vi "test1-TestModuleStatusVI.vi"(8 "error in (no error)":errorcluster, 11 "TestCase in":refnum<class "testcase-CSMManagementAPI.lvclass">) -> (0 "error out":errorcluster, 3 "TestCase out":refnum<class "testcase-CSMManagementAPI.lvclass">)   [LabVIEW 2017, in "testcase-CSMManagementAPI.lvclass"]
uses:
  testcase-CSMManagementAPI.lvclass
  src/user.lib/_NEVSTOP/Communicable State Machine(CSM)/_Support/Typedef/_CSM_MODE.ctl
  src/user.lib/_NEVSTOP/Communicable State Machine(CSM)/AdvanceAPI/CSM - Revert Arguments-Safe String.vi
  src/user.lib/_NEVSTOP/Communicable State Machine(CSM)/AdvanceAPI/CSM - Make String Arguments Safe.vi
  src/user.lib/_NEVSTOP/Communicable State Machine(CSM)/AdvanceAPI/CSM - Break Down Multiple States String.vi
  src/user.lib/_NEVSTOP/Communicable State Machine(CSM)/AdvanceAPI/CSM - Compact Multiple States.vi
  src/user.lib/_NEVSTOP/Communicable State Machine(CSM)/AdvanceAPI/CSM - Keywords.vi
  src/user.lib/_NEVSTOP/Communicable State Machine(CSM)/_Shared/Trim Single-line Text.vi
  <vilib>/addons/_JKI Toolkits/VI Tester/TestCase.llb/TestCase.lvclass
  src/user.lib/_NEVSTOP/Communicable State Machine(CSM)/Communicable State Machine.lvlib
  src/user.lib/_NEVSTOP/Communicable State Machine(CSM)/_Support/Typedef/_CSM_List Module Scope.ctl
  CSM/CSM-Testcase.lvlib
  C:/Program Files (x86)/National Instruments/LabVIEW 2017/vi.lib/addons/_JKI Toolkits/VI Tester/TestCase.llb/TestCase.lvclass
panel:
  out "State History":string
  out "LoopCount":i32
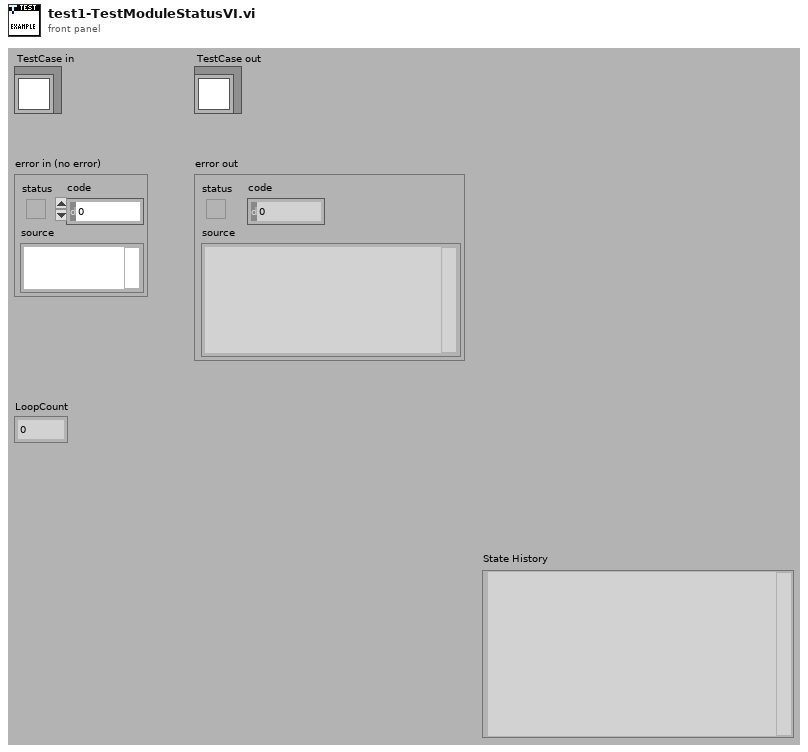
[diagram p1: front panel]
types:
  T1 = typedef "Communicable State Machine.lvlib/_CSM_MODE.ctl" = enum16{"Not Exist", "Stand Alone", "CSM", "Worker", "Worker Agent", "Chain Node", "Chain"}
  T2 = cluster{"CSM Name (Dup)":string, "Mode":T1, "#Nodes":i32}[]
  T3 = typedef "Communicable State Machine.lvlib/_CSM_List Module Scope.ctl" = enum16{"Normal", "System Only", "All"}
  T4 = enum32{"Invalid", "Standard", "Closed", "Hidden", "Minimized", "Maximized"}
  T5 = enum32{"invalid app kind", "Development System", "Run Time System", "Student Edition", "Embedded LabVIEW", "Evaluation", "Custom"}
  T6 = typedef "Communicable State Machine.lvlib/_CSM_Response Source Message.ctl" = cluster{"‘State":string, "’Arguments":string, "’Error":errorcluster}
  T7 = cluster{"Current VI Reference":refnum<vi>, "Close Panel on Exit?":bool}
  T8 = cluster{"Core":cluster{"Current VI Reference":refnum<vi>, "Close Panel on Exit?":bool}, "Your Boolean data":bool, "Your string data":string, "Module Status":cluster{"CSM Name (Dup)":string, "Mode":T1, "#Nodes":i32}}
  T9 = cluster{"CSM Name (Dup)":string, "Mode":T1, "#Nodes":i32}
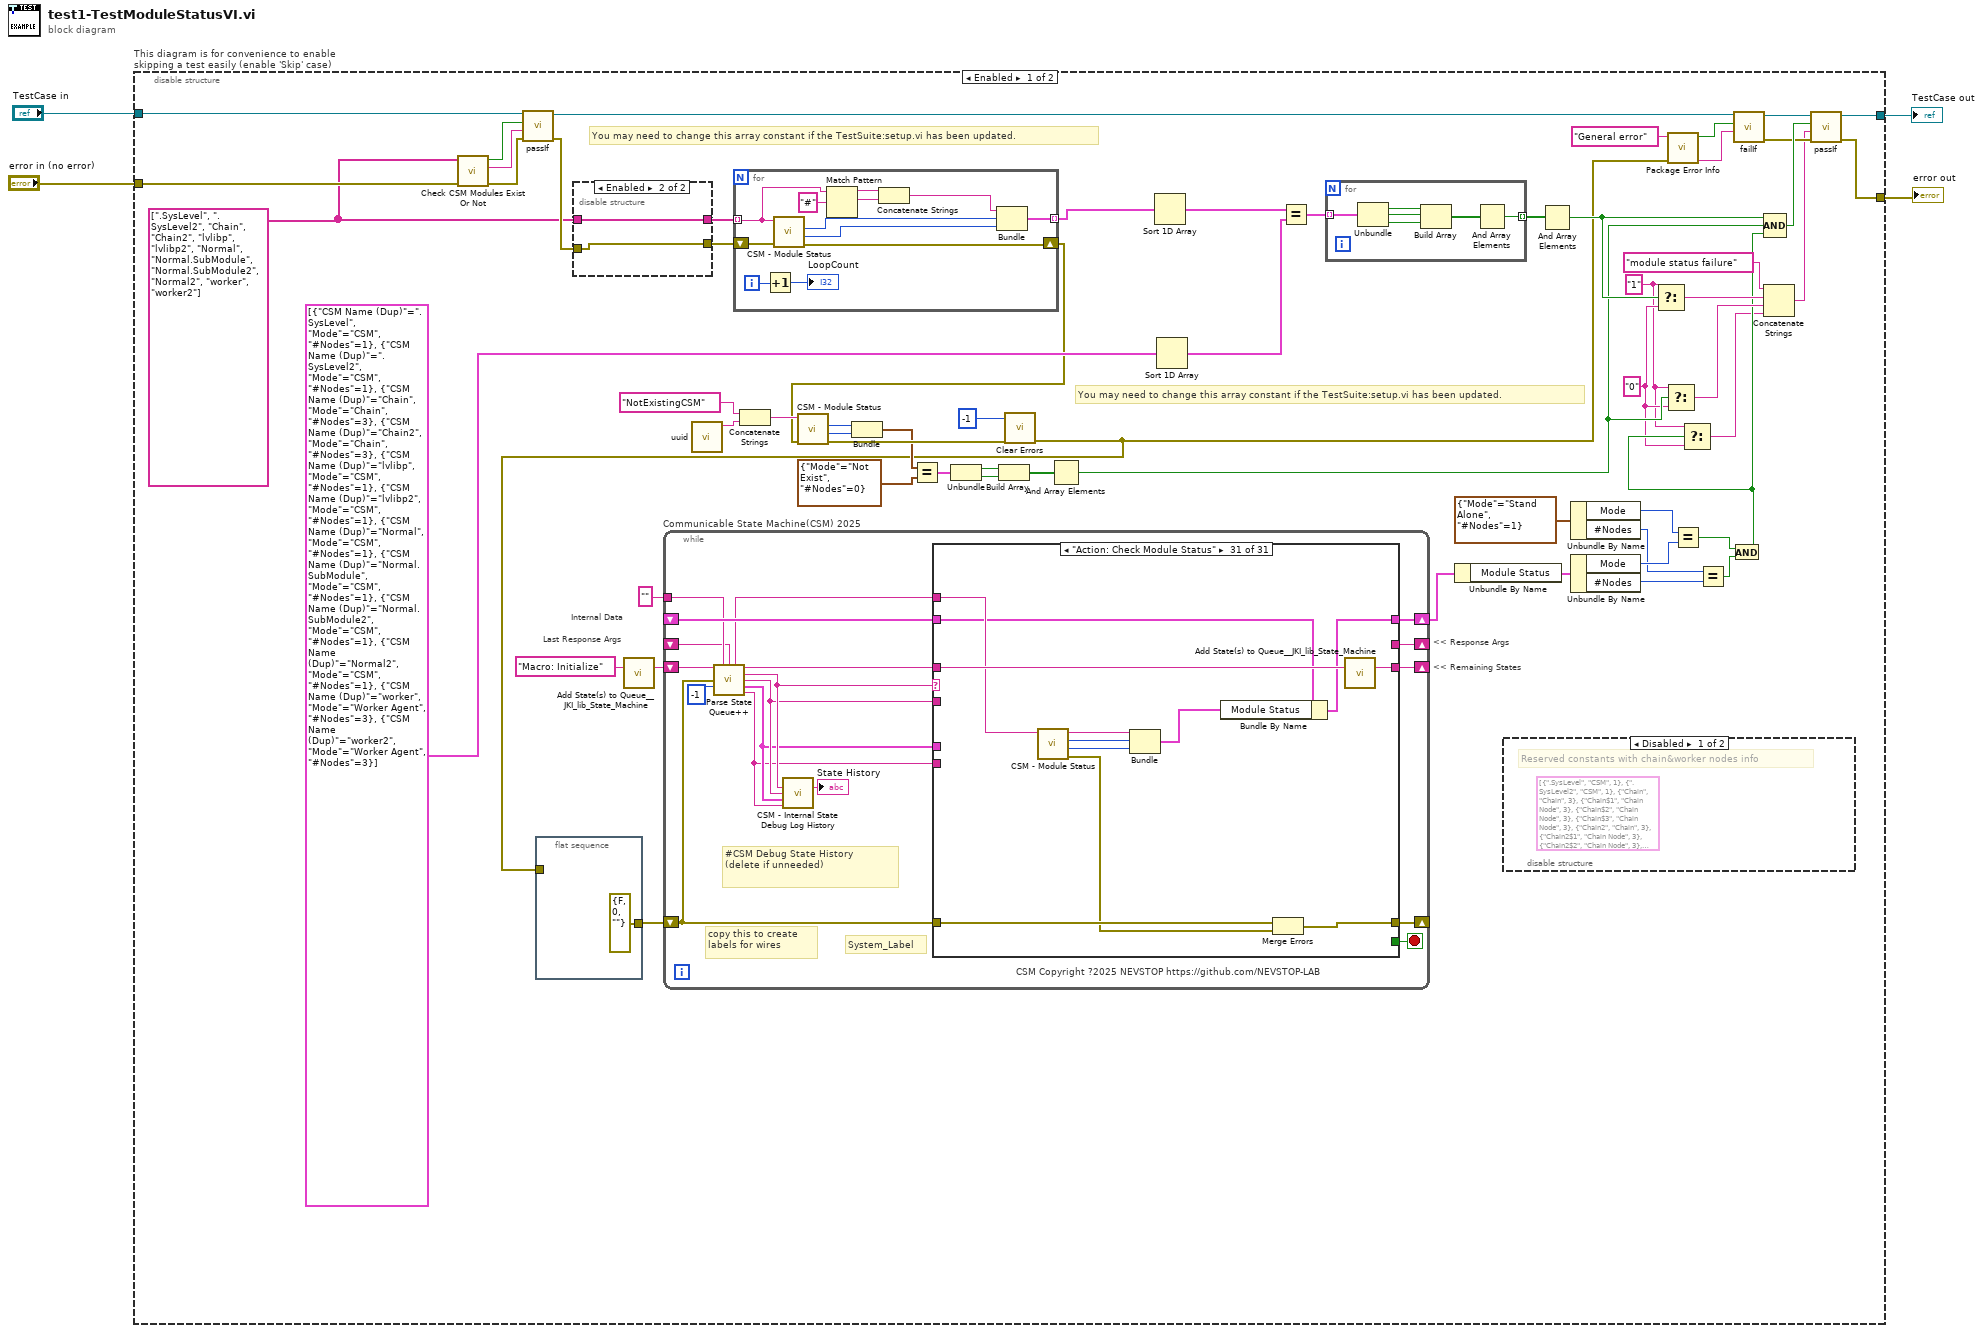
[diagram p0: block diagram]
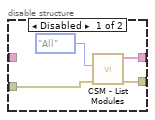
[diagram p3: hidden frame]
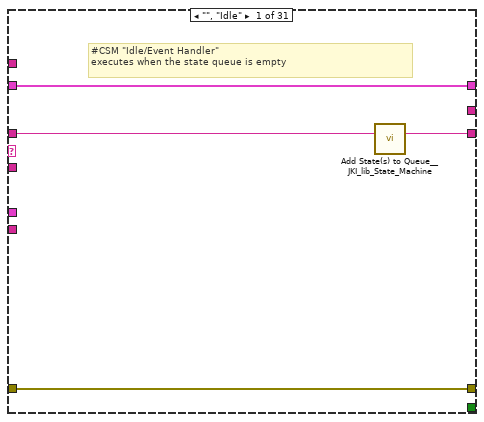
[diagram p4: hidden frame]
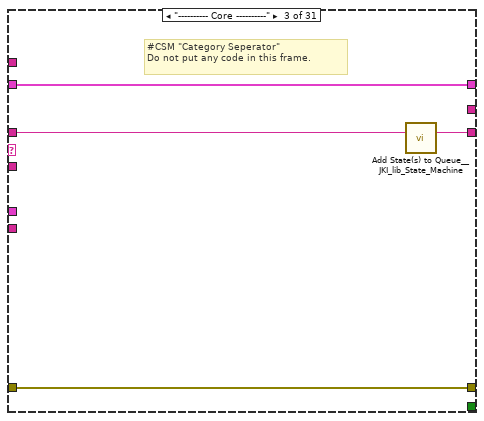
[diagram p6: hidden frame]
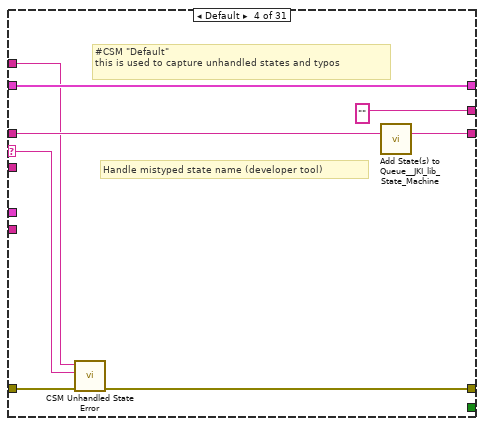
[diagram p7: hidden frame]
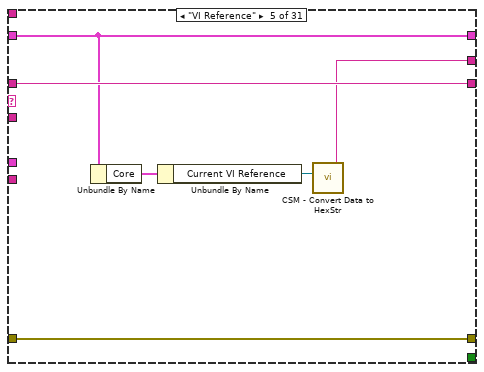
[diagram p8: hidden frame]
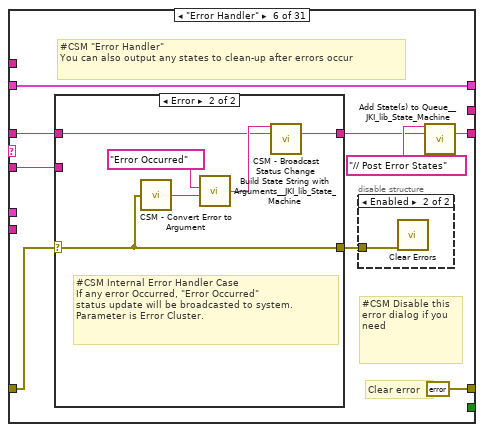
[diagram p9: hidden frame]
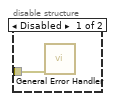
[diagram p10: hidden frame]
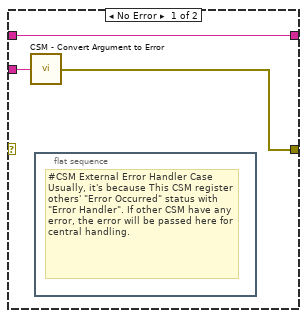
[diagram p11: hidden frame]
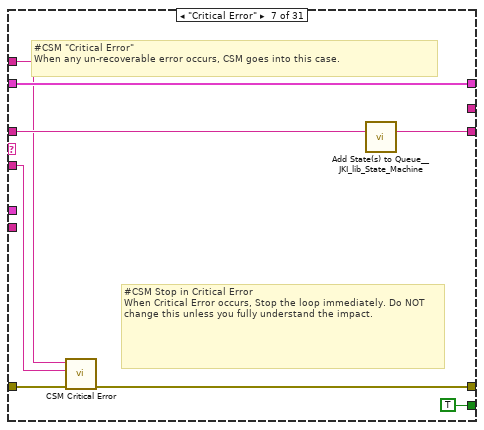
[diagram p12: hidden frame]
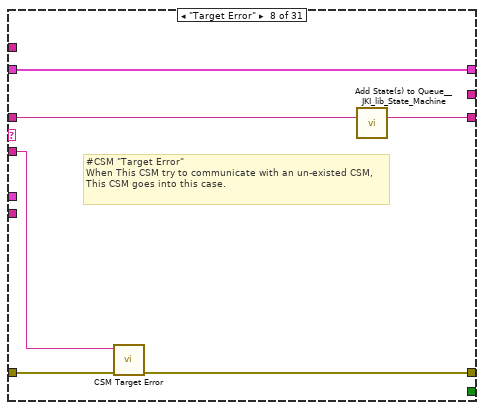
[diagram p13: hidden frame]
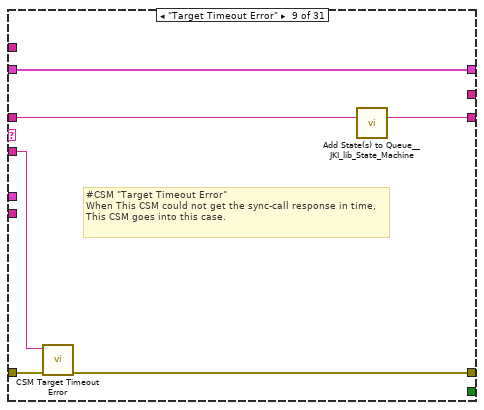
[diagram p14: hidden frame]
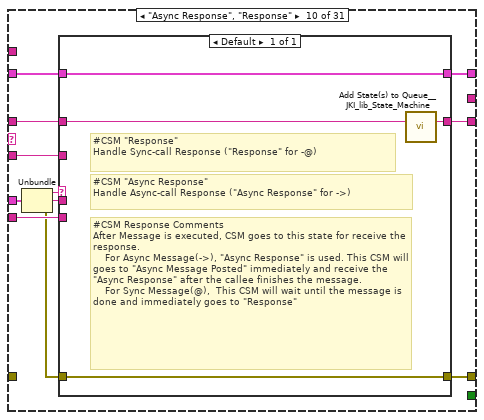
[diagram p15: hidden frame]
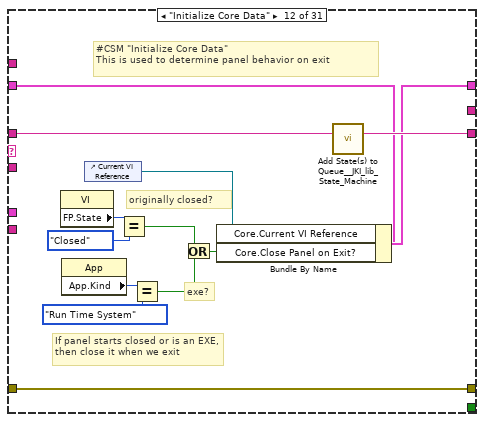
[diagram p17: hidden frame]
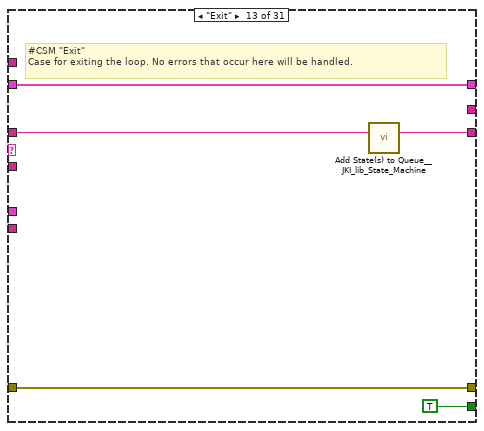
[diagram p18: hidden frame]
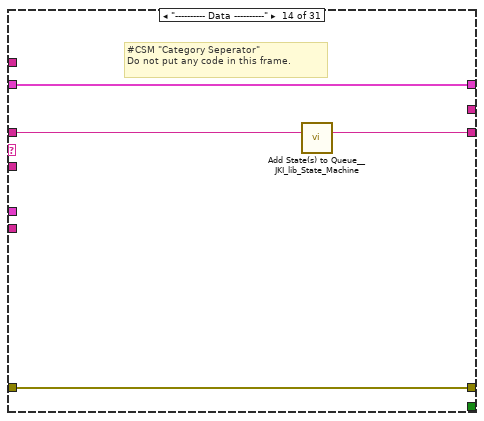
[diagram p19: hidden frame]
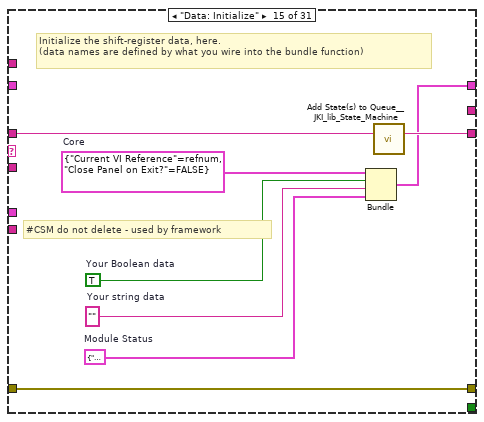
[diagram p20: hidden frame]
diagram:
  n1 = disable-structure "This diagram is for convenience to enable skipping a test easily (enable 'Skip' case)" shown="Enabled" {
    disable-tunnel: "TestCase in" -> [w26 w383]
    disable-tunnel: [w64 w381] -> w1
    disable-tunnel: [w63 w382] -> w3
    disable-tunnel: "error in (no error)" -> [w25 w380]
    frame Enabled {
      w11 = "0" ("f")
      w10 = "1"
      w5 = string[] [".SysLevel", ".SysLevel2", "Chain", "Chain2", "lvlibp", "lvlibp2", "Normal", "Normal.SubModule", "Normal.SubModule2", "Normal2", "worker", "worker2"] ("Module Names in All Scope")
      # "You may need to change this array constant if the TestSuite:setup.vi has been updated."
      # "You may need to change this array constant if the TestSuite:setup.vi has been updated."
      # "Last Response Args"
      # "Internal Data"
      # "<< Response Args"
      # "<< Remaining States"
      n2 = call "Check CSM Modules Exist Or Not.vi"("error in"=w25, "CSM names in"=w5) -> ("error out"=w27:errorcluster, "Debug string"=w28:string, "All Modules Exist?"=w29:bool)  [unwired: 7 in]
      n3 = call-dynamic "passIf.vi"("error in (no error)"=w27, "message (\"\")"=w28, "pass"=w29, "TestCase in"=w26) -> ("error out"=w24:errorcluster, "TestCase out"=w21:refnum<class "testcase-CSMManagementAPI.lvclass">)  [unwired: 6 in]
      n4 = flat-sequence {
        tunnel: [errorcluster {"status"=FALSE, "code"=0, "source"=""} ("error out")] -> w62
        tunnel: w6 -> [_]
        frame #0 {
        }
      }
      n5 = disable-structure shown="Enabled" {
        disable-tunnel: [w69 w72] -> w66
        disable-tunnel: [w68 w71] -> w65
        disable-tunnel: w24 -> [w67 w72]
        disable-tunnel: w5 -> [_ w71]
        frame Disabled {
          n6 = call "CSM - List Modules.vi"("Error In"=w67, "Scope (Normal)"=_CSM_List_Module_Scope."All") -> ("error out"=w69:errorcluster, "Module Names"=w68:string[])  [unwired: 8 in]
        }
        frame Enabled {
        }
      }
      n7 = call <vilib>:"Add State(s) to Queue__JKI_lib_State_Machine.vi"("State(s) in (\"\")"="Macro: Initialize" ("Init State(\"Macro: Initialize\")")) -> ("States Out"=w59:string)  [unwired: 14 in]
      n8 = while "Communicable State Machine(CSM) 2025" {
        shift-right: [w92] -> w58
        shift-left: _ -> [w91]
        shift-right: [w95] -> _
        shift-left: w62 -> [w90]
        shift-right: [w94] -> _
        shift-left: w59 -> [w96]
        tunnel: "" ("Name (\"\" to Use UUID)") -> [w88]
        shift-right: [w89] -> _
        shift-left: _ -> [w82]
        stop <- w93 stop-if-true
        # "#CSM Debug State History\n(delete if unneeded)"
        # "copy this to create labels for wires"
        # "System_Label"
        # "CSM Copyright ?2025 NEVSTOP https://github.com/NEVSTOP-LAB"
        n9 = call "Parse State Queue++.vi"("State Queue"=w96, "Name (\"\" to Use UUID)"=w88, "Response Arguments"=w82, "Previous Error"=w90, "Dequeue (1 ms)"=-1 ("Timeout")) -> ("Name Used"=w83:string, "Remaining States"=w97:string, "Current State"=w87:string, "Arguments"=w86:string, "Additional Information"=w85:T6, "Source CSM"=w84:string)  [unwired: 5 in]
        n10 = call "CSM - Internal State Debug Log History.vi"("State"=w87, "Arguments (\"\")"=w86, ">> Response Source Message >>"=w85, "Source (\"\")"=w84) -> ("Debug Log"=→"State History":string)  [unwired: 11 in]
        n11 = case shown="\"Action: Check Module Status\"" w87 {
          selector: w87 -> [_ _ _ w111 _ _ _ _ _ _ _ _ _ _ _ _ _ _ _ _ _ _ _ _ _ _ _ _ _ _ _]
          tunnel: w97 -> [w98 w103 w108 w115 w121 w127 w148 w154 w160 w168 w179 w193 w198 w202 w210 w212 w219 w223 w227 w233 w248 w317 w322 w329 w331 w335 w340 w347 w351 w355 w367]
          tunnel: w86 -> [_ _ _ _ _ w126 w144 w153 w158 w167 _ _ _ _ _ _ _ _ _ w228 w242 _ _ _ _ _ w338 _ _ _ _]
          tunnel: w91 -> [w99 w102 w105 w113 w120 w130 w149 w155 w161 w170 w178 w186 w196 w199 _ w211 w214 w220 w225 w231 w244 w314 w319 w326 w330 w334 w339 w344 w348 w352 w360]
          tunnel: [w100 w104 w106 w109 w122 errorcluster {"status"=FALSE, "code"=0, "source"=""} ("error out") w145 w151 w157 w173 w180 w190 w195 w200 w207 w213 w215 w221 w224 w229 w245 w315 w320 w327 w332 w336 w341 w345 w349 w353 w357] -> w95
          tunnel: w90 -> [w100 w104 w106 w116 w122 w128 w150 w152 w159 _ w180 w190 w195 w200 w207 w213 w216 w221 w224 w230 w246 w315 w320 w327 w332 w336 w341 w345 w349 w353 w365]
          tunnel: [w101 w103 w107 w114 w121 w123 w147 w156 w162 w169 w179 w192 w197 w201 w209 w212 w218 w222 w226 w232 w247 w316 w321 w328 w331 w335 w340 w346 w350 w354 w366] -> w94
          tunnel: [_ _ _ _ _ _ TRUE _ _ _ _ _ TRUE _ _ _ _ _ _ _ _ _ _ _ _ _ _ _ _ _ _] -> w93
          tunnel: [w99 w102 w105 w113 w120 w130 w149 w155 w161 w171 w178 w191 w196 w199 w208 w211 w214 w220 w225 w231 w244 w314 w319 w326 w330 w334 w339 w344 w348 w352 w359] -> w92
          tunnel: w84 -> [_ _ _ _ _ _ _ _ _ w165 _ _ _ _ _ _ _ _ _ _ _ _ _ _ _ _ _ _ _ _ _]
          tunnel: w85 -> [_ _ _ _ _ _ _ _ _ w172 _ _ _ _ _ _ _ _ _ _ _ _ _ _ _ _ _ _ _ _ _]
          tunnel: [_ _ _ "" w117 _ _ _ _ _ _ _ _ _ _ _ _ _ _ _ _ _ _ _ _ "API1 Response" w337 _ _ _ _] -> w89
          tunnel: w83 -> [_ _ _ w110 _ _ w143 _ _ _ _ _ _ _ _ _ _ _ _ _ _ _ _ _ _ _ _ _ _ _ w364]
          frame "", "Idle" {
            # "#CSM \"Idle/Event Handler\"\nexecutes when the state queue is empty"
            n12 = call <vilib>:"Add State(s) to Queue__JKI_lib_State_Machine.vi"("State(s) in (\"\")"=w98) -> ("States Out"=w101:string)  [unwired: 14 in]
          }
          frame "CSM Documentation" {
            # "#CSM README FIRST\n\nCommunicable State Machine(CSM) is a LabVIEW application framework that builds upon JKI State Machine(JKISM). It follows the pattern of JKISM and extends the keywords to describe message communication between modules, including concepts such as Sync-Message, Async-Message, Subscription/Unsubscription of status - essential elements for creating reusable code modules. For more information, please visit the CSM wiki: https://nevstop-lab.github.io/CSM-Wiki/\n\nFor instructions on JKI State Machine, visit: http://jki.net/state-machine/\nFor information about CSM, visit: https://github.com/NEVSTOP-LAB"
            # "#CSM \"Documentation\"\nCase for holding CSM Documenation"
          }
          frame "---------- Core ----------" {
            # "#CSM \"Category Seperator\"\nDo not put any code in this frame."
            n13 = call <vilib>:"Add State(s) to Queue__JKI_lib_State_Machine.vi"("State(s) in (\"\")"=w108) -> ("States Out"=w107:string)  [unwired: 14 in]
          }
          frame Default {
            # "#CSM \"Default\"\nthis is used to capture unhandled states and typos"
            # "Handle mistyped state name (developer tool)"
            n14 = call "CSM Unhandled State Error.vi"("error in (no error)"=w116, "Undefined State"=w111, "CSM Name"=w110) -> ("error out"=w109:errorcluster)  [unwired: 8 in]
            n15 = call <vilib>:"Add State(s) to Queue__JKI_lib_State_Machine.vi"("State(s) in (\"\")"=w115) -> ("States Out"=w114:string)  [unwired: 14 in]
          }
          frame "VI Reference" {
            n16 = Unbundle By Name(w120) -> ("Core"=w119:T7)
            n17 = Unbundle By Name(w119) -> ("Current VI Reference"=w118:refnum<vi>)
            n18 = call "CSM - Convert Data to HexStr.vi"("Variant"=w118) -> ("HEX String (0-9,A-F)"=w117:string)  [unwired: 8 in]
          }
          frame "Error Handler" {
            # "#CSM Disable this error dialog if you need"
            # "#CSM \"Error Handler\"\nYou can also output any states to clean-up after errors occur"
            # "Clear error"
            n19 = case shown="Error" w128 {
              selector: w128 -> [_ w137]
              tunnel: [w136 w139] -> w124
              tunnel: w127 -> [w136 w138]
              tunnel: w126 -> [w135 _]
              tunnel: [w134 w137] -> w129
              frame No Error {
                n20 = call "CSM - Convert Argument to Error.vi"("Argument"=w135) -> ("Error"=w134:errorcluster)  [unwired: 4 in]
                n21 = flat-sequence {
                  frame #0 {
                    # "#CSM External Error Handler Case\nUsually, it's because This CSM register others' \"Error Occurred\" status with \"Error Handler\". If other CSM have any error, the error will be passed here for central handling."
                  }
                }
              }
              frame Error {
                # "#CSM Internal Error Handler Case \nIf any error Occurred, \"Error Occurred\" \nstatus update will be broadcasted to system.\nParameter is Error Cluster."
                n22 = call "CSM - Convert Error to Argument.vi"("Error"=w137) -> ("Argument"=w141:string)  [unwired: 4 in]
                n23 = call <vilib>:"Build State String with Arguments__JKI_lib_State_Machine.vi"("Arguments (\"\")"=w141, "State"="Error Occurred" ("Status with Arguments")) -> ("State with Arguments"=w140:string)  [unwired: 4 in]
                n24 = call "CSM - Broadcast Status Change.vi"("Status With Arguments"=w140, "State Queue"=w138) -> ("Remaining States"=w139:string)  [unwired: 13 in]
              }
            }
            n25 = disable-structure shown="Enabled" {
              disable-tunnel: w129 -> [w132 w133]
              frame Disabled {
                n26 = call <vilib>:"General Error Handler.vi"("error in (no error)"=w132) -> ()  [unwired: 10 in, 5 out]
              }
              frame Enabled {
                n27 = call <vilib>:"Clear Errors.vi"("error in (no error)"=w133) -> ()  [unwired: 5 in, 2 out]
              }
            }
            n28 = call <vilib>:"Add State(s) to Queue__JKI_lib_State_Machine.vi"("State(s) in Front (\"\")"="// Post Error States", "State(s) in (\"\")"=w124) -> ("States Out"=w123:string)  [unwired: 13 in]
          }
          frame "Critical Error" {
            # "#CSM Stop in Critical Error\nWhen Critical Error occurs, Stop the loop immediately. Do NOT change this unless you fully understand the impact."
            # "#CSM \"Critical Error\"\nWhen any un-recoverable error occurs, CSM goes into this case."
            n29 = call "CSM Critical Error.vi"("error in (no error)"=w150, "Arugments (As Reason)"=w144, "CSM Name"=w143) -> ("error out"=w145:errorcluster)  [unwired: 8 in]
            n30 = call <vilib>:"Add State(s) to Queue__JKI_lib_State_Machine.vi"("State(s) in (\"\")"=w148) -> ("States Out"=w147:string)  [unwired: 14 in]
          }
          frame "Target Error" {
            # "#CSM \"Target Error\"\nWhen This CSM try to communicate with an un-existed CSM, This CSM goes into this case."
            n31 = call "CSM Target Error.vi"("error in (no error)"=w152, "Arguments (As CSM Name)"=w153) -> ("error out"=w151:errorcluster)  [unwired: 9 in]
            n32 = call <vilib>:"Add State(s) to Queue__JKI_lib_State_Machine.vi"("State(s) in (\"\")"=w154) -> ("States Out"=w156:string)  [unwired: 14 in]
          }
          frame "Target Timeout Error" {
            # "#CSM \"Target Timeout Error\"\nWhen This CSM could not get the sync-call response in time, This CSM goes into this case."
            n33 = call "CSM Target Timeout Error.vi"("error in (no error)"=w159, "Arguments (As CSM Name)"=w158) -> ("error out"=w157:errorcluster)  [unwired: 9 in]
            n34 = call <vilib>:"Add State(s) to Queue__JKI_lib_State_Machine.vi"("State(s) in (\"\")"=w160) -> ("States Out"=w162:string)  [unwired: 14 in]
          }
          frame "Async Response", "Response" {
            n35 = Unbundle(w172) -> ("‘State"=w166:string, "’Arguments"=w164:string, "’Error"=w163:errorcluster)
            n36 = case shown="Default" w166 {
              tunnel: [w177] -> w173
              tunnel: w163 -> [w177]
              tunnel: [w176] -> w171
              tunnel: w170 -> [w176]
              tunnel: [w174] -> w169
              tunnel: w168 -> [w175]
              tunnel: w167 -> [_]
              tunnel: w165 -> [_]
              tunnel: w164 -> [_]
              frame Default {
                # "#CSM Response Comments\nAfter Message is executed, CSM goes to this state for receive the response.\n    For Async Message(->), \"Async Response\" is used. This CSM will goes to \"Async Message Posted\" immediately and receive the \"Async Response\" after the callee finishes the message.\n    For Sync Message(@),  This CSM will wait until the message is done and immediately goes to \"Response\""
                # "#CSM \"Async Response\"\nHandle Async-call Response (\"Async Response\" for ->)"
                # "#CSM \"Response\"\nHandle Sync-call Response (\"Response\" for -@)"
                n37 = call <vilib>:"Add State(s) to Queue__JKI_lib_State_Machine.vi"("State(s) in (\"\")"=w175) -> ("States Out"=w174:string)  [unwired: 14 in]
              }
            }
          }
          frame "Async Message Posted" {
            # "#CSM \"Async Message Posted\"\nAfter Async Message is posted (-> or ->| ), CSM goes to this state for post-action.\nYou can use Argument - State to tell which Async Message is called."
          }
          frame "Initialize Core Data" {
            # "#CSM \"Initialize Core Data\"\nThis is used to determine panel behavior on exit"
            # "originally closed?"
            # "exe?"
            # "If panel starts closed or is an EXE, then close it when we exit"
            n38 = property class="VI"() -> ("FP.State"=w183:T4)  [unwired: 2 in, 2 out]
            n39 = property class="App"() -> ("App.Kind"=w189:T5)  [unwired: 2 in, 2 out]
            n40 = control-ref of="Current VI Reference"() -> (w184:refnum<vi>)
            n41 = Equal?(x=w183, y=T4."Closed" ("Front Panel Window:State")) -> (x = y?=w181:bool)
            n42 = Equal?(x=w189, y=T5."Run Time System" ("Application:Kind")) -> (x = y?=w187:bool)
            n43 = Or(x=w181, y=w187) -> (x .or. y?=w185:bool)
            n44 = Bundle By Name(cluster=w186, "Core.Current VI Reference"=w184, "Core.Close Panel on Exit?"=w185) -> (w191:T8)
            n45 = call <vilib>:"Add State(s) to Queue__JKI_lib_State_Machine.vi"("State(s) in (\"\")"=w193) -> ("States Out"=w192:string)  [unwired: 14 in]
          }
          frame "Exit" {
            # "#CSM \"Exit\"\nCase for exiting the loop. No errors that occur here will be handled."
            n46 = call <vilib>:"Add State(s) to Queue__JKI_lib_State_Machine.vi"("State(s) in (\"\")"=w198) -> ("States Out"=w197:string)  [unwired: 14 in]
          }
          frame "---------- Data ----------" {
            # "#CSM \"Category Seperator\"\nDo not put any code in this frame."
            n47 = call <vilib>:"Add State(s) to Queue__JKI_lib_State_Machine.vi"("State(s) in (\"\")"=w202) -> ("States Out"=w201:string)  [unwired: 14 in]
          }
          frame "Data: Initialize" {
            w203 = T9 {"CSM Name (Dup)"="", "Mode"=enum."Not Exist", "#Nodes"=0}  # Module Status
            w204 = T7 {"Current VI Reference"=refnum, "Close Panel on Exit?"=FALSE}  # Core
            w206 = TRUE  # Your Boolean data
            w205 = ""  # Your string data
            # "#CSM do not delete - used by framework"
            # "Initialize the shift-register data, here.\n(data names are defined by what you wire into the bundle function)"
            n48 = Bundle("Core"=w204, "Your Boolean data"=w206, "Your string data"=w205, "Module Status"=w203) -> (w208:T8)  [unwired: 1 in]
            n49 = call <vilib>:"Add State(s) to Queue__JKI_lib_State_Machine.vi"("State(s) in (\"\")"=w210) -> ("States Out"=w209:string)  [unwired: 14 in]
          }
          frame "Data: Update Indicators" {
          }
          frame "Data: Cleanup" {
            # "Cleanup any data and references, here.\n(this is called automatically, by the Macro: Exit)"
            n50 = Unbundle By Name(w214) -> ("Core.Current VI Reference"=w217:refnum<vi>)
            n51 = Close Reference(reference=w217, error in (no error)=w216) -> (error out=w215:errorcluster)
            n52 = call <vilib>:"Add State(s) to Queue__JKI_lib_State_Machine.vi"("State(s) in (\"\")"=w219) -> ("States Out"=w218:string)  [unwired: 14 in]
          }
          frame "---------- UI ----------" {
            # "#CSM \"Category Seperator\"\nDo not put any code in this frame."
            n53 = call <vilib>:"Add State(s) to Queue__JKI_lib_State_Machine.vi"("State(s) in (\"\")"=w223) -> ("States Out"=w222:string)  [unwired: 14 in]
          }
          frame "UI: Initialize" {
            # "#CSM \"UI: Initialize\"\nInitialize the User Interface, here.\n(this is called automatically, by the Macro: Init)"
            n54 = call <vilib>:"Add State(s) to Queue__JKI_lib_State_Machine.vi"("State(s) in (\"\")"=w227) -> ("States Out"=w226:string)  [unwired: 14 in]
          }
          frame "UI: Cursor Set" {
            # "#CSM \"UI: Cursor Set\"\nSet and Unset Cursor Busy.\n(Usage: \"UI: Cursor Set >> Busy|Idle\")"
            # "Argument"
            n55 = disable-structure shown="TARGET_TYPE!=Windows" {
              disable-tunnel: w230 -> [w236 w241]
              disable-tunnel: [w235 w241] -> w229
              disable-tunnel: w228 -> [w234 _]
              frame condition #0 (active) {
                n56 = case shown="\"Idle\", Default" w234 {
                  tunnel: w236 -> [w238 w240]
                  tunnel: [w237 w239] -> w235
                  frame "Idle", Default {
                    n57 = call <vilib>:"Unset Busy.vi"("error in (no error)"=w238) -> ("error out"=w237:errorcluster)  [unwired: 10 in]
                  }
                  frame "Busy" {
                    n58 = call <vilib>:"Set Busy.vi"("error in (no error)"=w240) -> ("error out"=w239:errorcluster)  [unwired: 9 in, 1 out]
                  }
                }
              }
              frame condition #1 {
              }
            }
            n59 = call <vilib>:"Add State(s) to Queue__JKI_lib_State_Machine.vi"("State(s) in (\"\")"=w233) -> ("States Out"=w232:string)  [unwired: 14 in]
          }
          frame "UI: Front Panel State" {
            # "#CSM \"UI: Front Panel State\"\nSet Front Panel Open or Closed\n(Usage: \"UI: Front Panel State >> Open|Close\")"
            # "Argument"
            n60 = Unbundle By Name(w244) -> ("Core.Current VI Reference"=w243:refnum<vi>)
            n61 = call <vilib>:"Add State(s) to Queue__JKI_lib_State_Machine.vi"("State(s) in (\"\")"=w248) -> ("States Out"=w247:string)  [unwired: 14 in]
            n62 = case shown="\"Close\", \"Closed\"" w242 {
              tunnel: w246 -> [w254 w269 w280 w293 w306]
              tunnel: [w256 w270 w282 w295 w308] -> w245
              tunnel: w243 -> [w255 w267 w281 w294 w307]
              frame "Open", "Standard", Default {
                w249 = T4."Standard" ("State")
                n63 = property class="VI"(reference=w255, error in=w254) -> (reference out=w252:refnum<vi>, error out=w253:errorcluster, "FP.State"=w251:T4)
                n64 = Not Equal?(x=w251, y=w249) -> (x != y?=w250:bool)
                n65 = case shown="True" w250 {
                  tunnel: [w260 w262] -> w256
                  tunnel: w253 -> [w259 w262]
                  tunnel: w252 -> [w258 _]
                  tunnel: w249 -> [w257 _]
                  frame True {
                    n66 = invoke class="VI" method="FP.Open"(reference=w258, error in=w259, "Activate"=TRUE, "State"=w257) -> (error out=w260:errorcluster)  [unwired: 1 in, 4 out]
                  }
                  frame False {
                  }
                }
              }
              frame "Close", "Closed" {
                n67 = property class="VI"(reference=w267, error in=w269) -> (reference out=w266:refnum<vi>, error out=w268:errorcluster, "FP.State"=w264:T4)
                n68 = Not Equal?(x=w264, y=T4."Closed" ("Front Panel Window:State")) -> (x != y?=w263:bool)
                n69 = case shown="False" w263 {
                  tunnel: [w271 w274] -> w270
                  tunnel: w268 -> [w271 w273]
                  tunnel: w266 -> [_ w272]
                  frame False {
                  }
                  frame True {
                    n70 = invoke class="VI" method="FP.Close"(reference=w272, error in=w273) -> (error out=w274:errorcluster)  [unwired: 1 in, 2 out]
                  }
                }
              }
              frame "Hidden", "Hide" {
                w275 = T4."Hidden" ("State")
                n71 = property class="VI"(reference=w281, error in=w280) -> (reference out=w278:refnum<vi>, error out=w279:errorcluster, "FP.State"=w277:T4)
                n72 = Not Equal?(x=w277, y=w275) -> (x != y?=w276:bool)
                n73 = case shown="True" w276 {
                  tunnel: [w286 w287] -> w282
                  tunnel: w279 -> [w285 w287]
                  tunnel: w278 -> [w284 _]
                  tunnel: w275 -> [w283 _]
                  frame True {
                    n74 = invoke class="VI" method="FP.Open"(reference=w284, error in=w285, "State"=w283) -> (error out=w286:errorcluster)  [unwired: 2 in, 4 out]
                  }
                  frame False {
                  }
                }
              }
              frame "Minimize", "Minimized" {
                w288 = T4."Minimized" ("State")
                n75 = property class="VI"(reference=w294, error in=w293) -> (reference out=w291:refnum<vi>, error out=w292:errorcluster, "FP.State"=w290:T4)
                n76 = Not Equal?(x=w290, y=w288) -> (x != y?=w289:bool)
                n77 = case shown="True" w289 {
                  tunnel: [w299 w300] -> w295
                  tunnel: w292 -> [w298 w300]
                  tunnel: w291 -> [w297 _]
                  tunnel: w288 -> [w296 _]
                  frame True {
                    n78 = invoke class="VI" method="FP.Open"(reference=w297, error in=w298, "State"=w296) -> (error out=w299:errorcluster)  [unwired: 2 in, 4 out]
                  }
                  frame False {
                  }
                }
              }
              frame "Maximize", "Maximized" {
                w301 = T4."Maximized" ("State")
                n79 = property class="VI"(reference=w307, error in=w306) -> (reference out=w304:refnum<vi>, error out=w305:errorcluster, "FP.State"=w303:T4)
                n80 = Not Equal?(x=w303, y=w301) -> (x != y?=w302:bool)
                n81 = case shown="True" w302 {
                  tunnel: [w312 w313] -> w308
                  tunnel: w305 -> [w311 w313]
                  tunnel: w304 -> [w310 _]
                  tunnel: w301 -> [w309 _]
                  frame True {
                    n82 = invoke class="VI" method="FP.Open"(reference=w310, error in=w311, "State"=w309) -> (error out=w312:errorcluster)  [unwired: 2 in, 4 out]
                  }
                  frame False {
                  }
                }
              }
            }
          }
          frame "---------- Macro ----------" {
            # "#CSM \"Category Seperator\"\nDo not put any code in this frame."
            n83 = call <vilib>:"Add State(s) to Queue__JKI_lib_State_Machine.vi"("State(s) in (\"\")"=w317) -> ("States Out"=w316:string)  [unwired: 14 in]
          }
          frame "Macro: Initialize" {
            # "#CSM \"Macro: Initialize\"\nInitialization Macro (This is called once, when the VI starts)"
            n84 = call <vilib>:"Add State(s) to Queue__JKI_lib_State_Machine.vi"("State(s) in Front (\"\")"="Data: Initialize\nInitialize Core Data\nData: Update Indicators\nAction: Check Module Status\nMacro: Exit", "State(s) in (\"\")"=w322) -> ("States Out"=w321:string)  [unwired: 13 in]
          }
          frame "Macro: Exit" {
            # "#CSM \"Macro: Exit\"\nExit Macro (This is called once, when the VI exits)"
            n85 = call <vilib>:"Add State(s) to Queue__JKI_lib_State_Machine.vi"("State(s) in Front (\"\")"="//Exit Sub-Modules ", "State(s) at Back (\"\")"="Data: Cleanup\nExit") -> ("States Out"=w324:string)  [unwired: 13 in]
            n86 = call <vilib>:"Add State(s) to Queue__JKI_lib_State_Machine.vi"("State(s) in Front (\"\")"=w324, "State(s) in (\"\")"=w329) -> ("States Out"=w328:string)  [unwired: 13 in]
          }
          frame "---------- API ----------" {
            # "#CSM \"Category Seperator\"\nDo not put any code in this frame."
          }
          frame "API: API1" {
            # "#CSM API Example\nCopy/Rename this case for your own API"
            # "#CSM Response\nConnect this to return the response of your API"
            # "#CSM >> Msg/Rep's CSM >>\nIf you need to tell who triggered this state , use this string. If it's this case itself, this string is \"\"."
            # "#CSM >> Arguments >>\nDeal with the parameter if any"
          }
          frame "API: API2" {
            # "#CSM API Example\nCopy/Rename this case for your own API"
            # "unpack Hex String  to Variant\nif complex parameter is needed."
            n87 = call "CSM - Convert HexStr to Data.vi"("HEX String"=w338) -> ()  [unwired: 7 in, 2 out]
            n88 = disable-structure shown="Disabled" {
              disable-tunnel: [w342 "API2 Response"] -> w337
              frame Disabled {
                # "pack variant to hexstr \nif complex response is needed."
                # "complex Response"
                n89 = call "CSM - Convert Data to HexStr.vi"() -> ("HEX String (0-9,A-F)"=w342:string)  [unwired: 9 in]
              }
              frame Enabled {
              }
            }
          }
          frame "---------- Action ----------" {
            # "#CSM \"Category Seperator\"\nDo not put any code in this frame."
            n90 = call <vilib>:"Add State(s) to Queue__JKI_lib_State_Machine.vi"("State(s) in (\"\")"=w347) -> ("States Out"=w346:string)  [unwired: 14 in]
          }
          frame "Action: action1" {
            # "#CSM \"Internal State\"\nThis category is used for holding internal states"
            n91 = call <vilib>:"Add State(s) to Queue__JKI_lib_State_Machine.vi"("State(s) in (\"\")"=w351) -> ("States Out"=w350:string)  [unwired: 14 in]
          }
          frame "Action: action2" {
            # "#CSM \"Internal State\"\nThis category is used for holding internal states"
            n92 = call <vilib>:"Add State(s) to Queue__JKI_lib_State_Machine.vi"("State(s) in (\"\")"=w355) -> ("States Out"=w354:string)  [unwired: 14 in]
          }
          frame "Action: Check Module Status" {
            n93 = call "CSM - Module Status.vi"("CSM Name"=w364) -> ("error out"=w356:errorcluster, "#Nodes"=w361:i32, "Mode"=w362:T1, "CSM Name (Dup)"=w363:string)  [unwired: 6 in, 1 out]
            n94 = Bundle("CSM Name (Dup)"=w363, "Mode"=w362, "#Nodes"=w361) -> (w358:T9)  [unwired: 1 in]
            n95 = Bundle By Name(cluster=w360, "Module Status"=w358) -> (w359:T8)
            n96 = Merge Errors(w365, w356) -> (w357:errorcluster)
            n97 = call <vilib>:"Add State(s) to Queue__JKI_lib_State_Machine.vi"("State(s) in (\"\")"=w367) -> ("States Out"=w366:string)  [unwired: 14 in]
          }
        }
      }
      n98 = call "uuid.vi"() -> ("UUID"=w52:string)  [unwired: 11 in]
      n99 = for {
        tunnel: w65 -> [w371] mode=indexing
        shift-right: [w378] -> w7
        shift-left: w66 -> [w379]
        tunnel: [w373] -> w50 mode=indexing
        i -> [w377]
        n100 = Increment(x=w377) -> (x+1=→"LoopCount":i32)
        n101 = call "CSM - Module Status.vi"("Error In"=w379, "CSM Name"=w371) -> ("error out"=w378:errorcluster, "#Nodes"=w374:i32, "Mode"=w375:T1)  [unwired: 5 in, 2 out]
        n102 = Match Pattern(string=w371, regular expression="#") -> (before substring=w370:string, match substring=w369:string)  [unwired: 1 in, 2 out]
        n103 = Concatenate Strings(w370, w369) -> (w368:string)
        n104 = Bundle(w368, "Mode"=w375, "#Nodes"=w374) -> (w373:cluster{string, "Mode":T1, "#Nodes":i32})  [unwired: 1 in]
      }
      n105 = Concatenate Strings("NotExistingCSM" ("CSM Name"), w52) -> (w51:string)
      n106 = call "CSM - Module Status.vi"("Error In"=w7, "CSM Name"=w51) -> ("error out"=w55:errorcluster, "#Nodes"=w56:i32, "Mode"=w57:T1)  [unwired: 5 in, 2 out]
      n107 = Bundle("Mode"=w57, "#Nodes"=w56) -> (w44:cluster{"Mode":T1, "#Nodes":i32})  [unwired: 1 in]
      n108 = Equal?(x=w44, y=cluster{"Mode":T1, "#Nodes":i32} {"Mode"=enum."Not Exist", "#Nodes"=0} ("Module Status")) -> (x = y?=w42:cluster{"Mode":bool, "#Nodes":bool})
      n109 = Unbundle(w42) -> ("Mode"=w41:bool, "#Nodes"=w40:bool)
      n110 = Build Array(w41, w40) -> (w39:bool[])
      n111 = call <vilib>:"Clear Errors.vi"("error in (no error)"=w55, "specific error code to clear (0: all)"=-1) -> ("error out"=w6:errorcluster)  [unwired: 4 in, 1 out]
      n112 = And Array Elements(Boolean array=w39) -> (logical AND=w14:bool)
      n113 = Sort 1D Array(array=w50) -> (sorted array=w48:cluster{string, "Mode":T1, "#Nodes":i32}[])
      n114 = Sort 1D Array(array=T2 [{"CSM Name (Dup)"=".SysLevel", "Mode"=enum."CSM", "#Nodes"=1}, {"CSM Name (Dup)"=".SysLevel2", "Mode"=enum."CSM", "#Nodes"=1}, {"CSM Name (Dup)"="Chain", "Mode"=enum."Chain", "#Nodes"=3}, {"CSM Name (Dup)"="Chain2", "Mode"=enum."Chain", "#Nodes"=3}, {"CSM Name (Dup)"="lvlibp", "Mode"=enum."CSM", "#Nodes"=1}, {"CSM Name (Dup)"="lvlibp2", "Mode"=enum."CSM", "#Nodes"=1}, {"CSM Name (Dup)"="Normal", "Mode"=enum."CSM", "#Nodes"=1}, {"CSM Name (Dup)"="Normal.SubModule", "Mode"=enum."CSM", "#Nodes"=1}, {"CSM Name (Dup)"="Normal.SubModule2", "Mode"=enum."CSM", "#Nodes"=1}, {"CSM Name (Dup)"="Normal2", "Mode"=enum."CSM", "#Nodes"=1}, {"CSM Name (Dup)"="worker", "Mode"=enum."Worker Agent", "#Nodes"=3}, {"CSM Name (Dup)"="worker2", "Mode"=enum."Worker Agent", "#Nodes"=3}] ("Module Status Array 2")) -> (sorted array=w47:T2)
      n115 = Equal?(x=w48, y=w47) -> (x = y?=w46:cluster{bool, "Mode":bool, "#Nodes":bool}[])
      n116 = for {
        tunnel: w46 -> [w79] mode=indexing
        tunnel: [w74] -> w45 mode=indexing
        n117 = Unbundle(w79) -> (w78:bool, "Mode"=w77:bool, "#Nodes"=w76:bool)
        n118 = Build Array(w78, w77, w76) -> (w75:bool[])
        n119 = And Array Elements(Boolean array=w75) -> (logical AND=w74:bool)
      }
      n120 = Unbundle By Name(w58) -> ("Module Status"=w38:T9)
      n121 = disable-structure shown="Disabled" {
        frame Disabled {
          (unwired) T2 [{"CSM Name (Dup)"=".SysLevel", "Mode"=enum."CSM", "#Nodes"=1}, {"CSM Name (Dup)"=".SysLevel2", "Mode"=enum."CSM", "#Nodes"=1}, {"CSM Name (Dup)"="Chain", "Mode"=enum."Chain", "#Nodes"=3}, {"CSM Name (Dup)"="Chain$1", "Mode"=enum."Chain Node", "#Nodes"=3}, {"CSM Name (Dup)"="Chain$2", "Mode"=enum."Chain Node", "#Nodes"=3}, {"CSM Name (Dup)"="Chain$3", "Mode"=enum."Chain Node", "#Nodes"=3}, {"CSM Name (Dup)"="Chain2", "Mode"=enum."Chain", "#Nodes"=3}, {"CSM Name (Dup)"="Chain2$1", "Mode"=enum."Chain Node", "#Nodes"=3}, {"CSM Name (Dup)"="Chain2$2", "Mode"=enum."Chain Node", "#Nodes"=3}, {"CSM Name (Dup)"="Chain2$3", "Mode"=enum."Chain Node", "#Nodes"=3}, {"CSM Name (Dup)"="lvlibp", "Mode"=enum."CSM", "#Nodes"=1}, {"CSM Name (Dup)"="lvlibp2", "Mode"=enum."CSM", "#Nodes"=1}, {"CSM Name (Dup)"="Normal", "Mode"=enum."CSM", "#Nodes"=1}, {"CSM Name (Dup)"="Normal.SubModule", "Mode"=enum."CSM", "#Nodes"=1}, {"CSM Name (Dup)"="Normal.SubModule2", "Mode"=enum."CSM", "#Nodes"=1}, {"CSM Name (Dup)"="Normal2", "Mode"=enum."CSM", "#Nodes"=1}, {"CSM Name (Dup)"="worker", "Mode"=enum."Worker Agent", "#Nodes"=3}, {"CSM Name (Dup)"="worker#", "Mode"=enum."Worker", "#Nodes"=3}, {"CSM Name (Dup)"="worker#", "Mode"=enum."Worker", "#Nodes"=3}, {"CSM Name (Dup)"="worker#", "Mode"=enum."Worker", "#Nodes"=3}, {"CSM Name (Dup)"="worker2", "Mode"=enum."Worker Agent", "#Nodes"=3}, {"CSM Name (Dup)"="worker2#", "Mode"=enum."Worker", "#Nodes"=3}, {"CSM Name (Dup)"="worker2#", "Mode"=enum."Worker", "#Nodes"=3}, {"CSM Name (Dup)"="worker2#", "Mode"=enum."Worker", "#Nodes"=3}] ("Module Status Array 2")
          # "Reserved constants with chain&worker nodes info"
        }
        frame Enabled {
        }
      }
      n122 = And Array Elements(Boolean array=w45) -> (logical AND=w16:bool)
      n123 = Unbundle By Name(cluster{"Mode":T1, "#Nodes":i32} {"Mode"=enum."Stand Alone", "#Nodes"=1} ("Module Status")) -> ("Mode"=w36:T1, "#Nodes"=w34:i32)
      n124 = Unbundle By Name(w38) -> ("Mode"=w35:T1, "#Nodes"=w33:i32)
      n125 = Select(t=w10, s=w16, f=w11) -> (s? t:f=w15:string)
      n126 = Select(t=w10, s=w14, f=w11) -> (s? t:f=w13:string)
      n127 = call "Package Error Info.vi"("error in"=w6, "String in"="General error") -> ("packed error info out"=w22:string, "error status"=w23:bool)  [unwired: 8 in]
      n128 = Equal?(x=w36, y=w35) -> (x = y?=w31:bool)
      n129 = Equal?(x=w34, y=w33) -> (x = y?=w32:bool)
      n130 = And(x=w31, y=w32) -> (x .and. y?=w12:bool)
      n131 = Select(t=w10, s=w12, f=w11) -> (s? t:f=w9:string)
      n132 = call-dynamic "failIf.vi"("message (\"\")"=w22, "fail"=w23, "TestCase in"=w21) -> ("error out"=w19:errorcluster, "TestCase out"=w20:refnum<class "testcase-CSMManagementAPI.lvclass">)  [unwired: 7 in]
      n133 = Compound Arithmetic op=AND(w16, w14, w12) -> (w30:bool)
      n134 = Concatenate Strings("module status failure" ("message (\"\")"), w15, w13, w9) -> (w8:string)
      n135 = call-dynamic "passIf.vi"("error in (no error)"=w19, "message (\"\")"=w8, "pass"=w30, "TestCase in"=w20) -> ("error out"=w63:errorcluster, "TestCase out"=w64:refnum<class "testcase-CSMManagementAPI.lvclass">)  [unwired: 6 in]
    }
    frame Disabled {
      # "skip test result while test is under development"
      n136 = call <vilib>:"skip.vi"("error in (no error)"=w380, "TestCase in"=w383) -> ("error out"=w382:errorcluster, "TestCase out"=w381:refnum<class "testcase-CSMManagementAPI.lvclass">)  [unwired: 8 in]
    }
  }
  "error out" <- w3
  "TestCase out" <- w1
